vi "Main.vi"(11 "Error in":errorcluster) -> (15 "Error out":errorcluster)   [LabVIEW 2020]
panel:
  out "Lavatory":string
  in  "stop":bool
  in  "Alarm Timer Limit":dbl
  out "Alarm Timer D":dbl
  out "Alarm Timer C":dbl
  out "Alarm Timer B":dbl
  out "Alarm Timer A":dbl
  in  "Lavatory D Occupied":bool
  in  "Lavatory B Occupied":bool
  in  "Lavatory C Occupied":bool
  in  "Lavatory A Occupied":bool
  in  "Alarm Acknowledge":bool
  in  "Seatbelt Sign ON":bool
  out "Alarm":bool
  out "Lavatories\nOccupied":bool
  out "Lavatories\nOccupied":bool
  out "Return to Seat":bool
  out "Return to Seat":bool
  out "Return to Seat":bool
  out "Return to Seat":bool
  out "Occupied":bool
  out "Occupied":bool
  out "Occupied":bool
  out "Occupied":bool
  # "Airplane Lavatory Signs"
  # "Front"
  # "Rear"
  # "Lavatory A"
  # "Lavatory C"
  # "Lavatory B"
  # "Lavatory D"
  # "Simulation Controls & Indicators"
  # "secs"
  # "secs"
  # "secs"
  # "secs"
  # "secs"
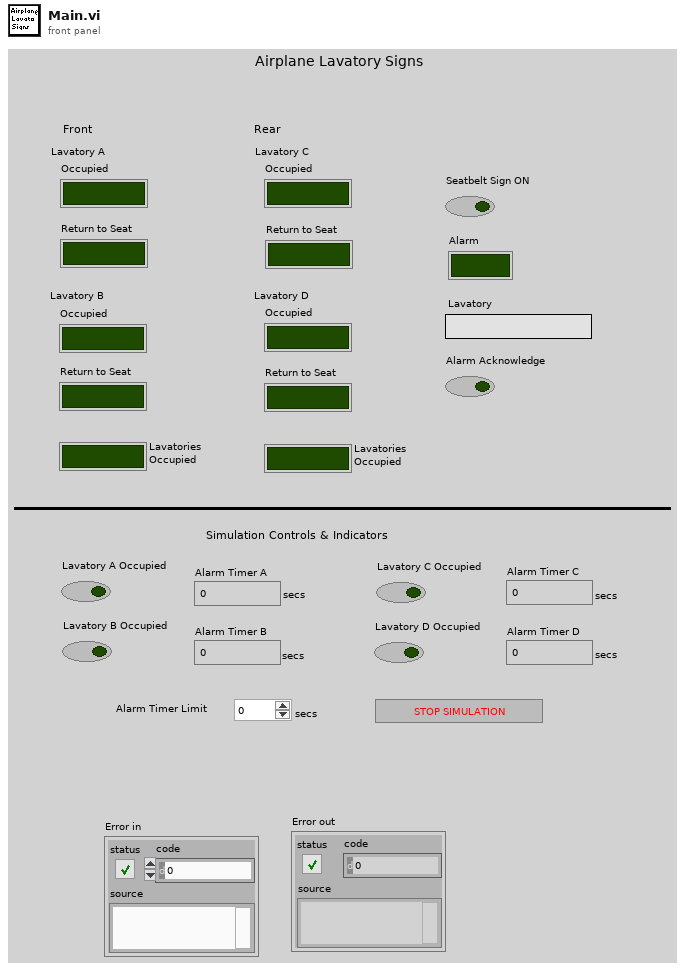
[diagram p1: front panel]
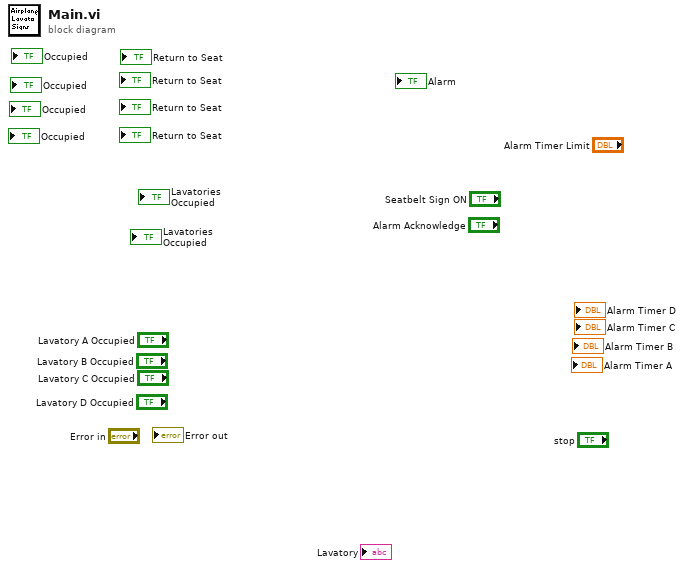
[diagram p0: block diagram]
diagram:
